vi "Door Open Interlock Value Change.vi"(8 "error in (no error)":errorcluster, 10 "Door Open Interlock":bool, 11 "Doors Closed in":refnum<class "Doors Closed.lvclass">) -> (0 "error out":errorcluster, 3 "Doors Closed out":refnum<class "Doors Closed.lvclass">)   [LabVIEW 2020, in "Door Controller.lvlib" / "Doors Closed.lvclass"]
uses:
  Doors Closed.lvclass
  C:/Users/Thomas.McQuillan/Desktop/Elevator Door Control/Door Controller/Door Controller/Door Controller.lvclass
  Application/Application/Interlock Names.ctl
  Door Controller/Door Controller.lvclass
  Application/Application.lvlib
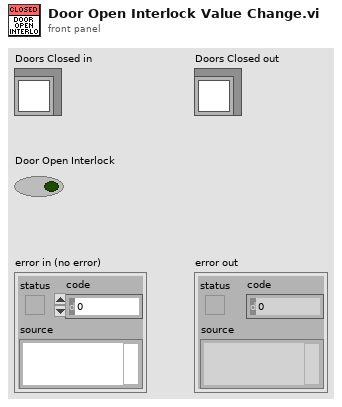
[diagram p1: front panel]
types:
  T1 = typedef "Application.lvlib/Interlock Names.ctl" = enum16{"Door Closed Interlock", "Door Open Interlock"}
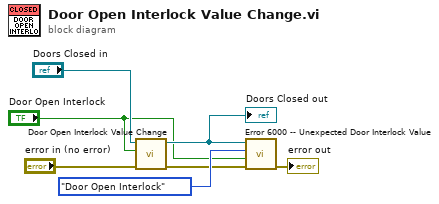
[diagram p0: block diagram]
diagram:
  n1 = call-parent "Door Open Interlock Value Change.vi"("error in (no error)"="error in (no error)", "Door Open Interlock"="Door Open Interlock", "Door Controller in"="Doors Closed in") -> ("error out"=w2:errorcluster, "Door Controller out"=w4:refnum<class "Doors Closed.lvclass">)  [unwired: 7 in]
  "Doors Closed out" <- w4
  n2 = call "Error 6000 -- Unexpected Door Interlock Value.vi"("error in (no error)"=w2, "Interlock Value"="Door Open Interlock", "Interlock Name"=Interlock_Names."Door Open Interlock", "Door Controller"=w4) -> ("error out"=→"error out":errorcluster)  [unwired: 7 in]
